vi "UHR-Fleezers Control (host) - 12.1_Jonathan.vi"() -> ()   [LabVIEW 2012] (continued)
            n1090 = Interleave 1D Arrays(w2555, w2554, w2553, w2538, w2552, w2551, w2501, w2521, w2520, w2500, w2519, w2518, w2523, w2522) -> (w2546:dbl[])
            n1091 = Divide(x=w2546, y=3276.7) -> (x/y=w2545:dbl[])
            n1092 = Decimate 1D Array(w2545) -> (w2544:dbl[], w2543:dbl[], w2542:dbl[], w2541:dbl[], w2540:dbl[], w2539:dbl[], w2497:dbl[], w2511:dbl[], w2495:dbl[], w2496:dbl[], w2509:dbl[], w2493:dbl[], w2507:dbl[], w2505:dbl[])
            n1093 = Negate(x=w2505) -> (-x=w2503:dbl[])
            n1094 = Divide(x=w2507, y=w2503) -> (x/y=w2506:dbl[])
            n1095 = Divide(x=w2496, y=w2493) -> (x/y=w2492:dbl[])
            n1096 = Divide(x=w2497, y=w2495) -> (x/y=w2494:dbl[])
            n1097 = Divide(x=w2544, y=w2542) -> (x/y=w2528:dbl[])
            n1098 = Divide(x=w2543, y=w2542) -> (x/y=w2527:dbl[])
            n1099 = Divide(x=w2541, y=w2539) -> (x/y=w2526:dbl[])
            n1100 = Divide(x=w2540, y=w2539) -> (x/y=w2525:dbl[])
            n1101 = Divide(x=w2511, y=w2495) -> (x/y=w2510:dbl[])
            n1102 = Divide(x=w2509, y=w2493) -> (x/y=w2508:dbl[])
            n1103 = Build Array(w2528, w2527, w2542, w2526, w2525, w2539, w2494, w2510, w2495, w2492, w2508, w2493, w2506, w2505) -> (w2504:dbl[][])
            n1104 = Bundle("T1 Y", "T1 X", "T1 Sum", "T2 Y", "T2 X", "T2 Sum", "T1 FB Y", "T1 FB X", "T1 FB Sum", "T2 FB Y", "T2 FB X", "T2 FB Sum", "PSD X", "PSD Y Sum") -> (w2491:T42)  [unwired: 1 out]
            n1105 = To Word Integer(number=w2546) -> (16bit integer=w2490:i16[])
            n1106 = Cluster To Array(cluster=w2491) -> (array=w2537:string[])
          }
        }
      }
    }
    "AI labels" <- w1624
    n1107 = Decimate 1D Array(w1598) -> (w1622:u32[], w1566:u32[])
    n1108 = local read "DMA Update Period (s)"() -> (w1634:dbl)
    n1109 = Build Array(w1622, w1566) -> (w1700:u32[][])
    n1110 = local read "Data Period (s)"() -> (w1472:dbl)
    n1111 = local read "BD 1 Frequency 2 (MHz)"() -> (w1505:dbl)
    n1112 = local read "BD 1 Frequency 1 (MHz)"() -> (w1506:dbl)
    n1113 = Decimate 1D Array(w1513) -> (w1537:i16[], w1536:i16[], w1534:i16[], w1533:i16[])  [unwired: 9 out]
    n1114 = To Double Precision Float(number=w1700) -> (double precision float=w1701:dbl[][])
    n1115 = local read "APD Integration Time (s)"() -> (w1579:dbl)
    n1116 = Multiply(x=w1472, y="Trap Pos. Disp. Downsample") -> (x*y=w1470:dbl)
    n1117 = Divide(x=w1537, y=w1536) -> (x/y=w1538:dbl[])
    n1118 = Divide(x=w1534, y=w1533) -> (x/y=w1535:dbl[])
    n1119 = feedback #6(0.0) -> (w1551:dbl)
    n1120 = Add(x=w1634, y=w1551) -> (x+y=w1740:dbl)
    n1121 = feedback-in #6(w1740) -> ()
    n1122 = local read "AOM X Cal (nm/MHz)"() -> (w1503:dbl)
    n1123 = To Time Stamp(1:w1551) -> (0:w1550:timestamp)
    n1124 = Split 1D Array(array=w1538, index="N El. to Ave.") -> (second subarray=w1541:dbl[])  [unwired: 1 out]
    n1125 = Split 1D Array(array=w1535, index="N El. to Ave.") -> (second subarray=w1540:dbl[])  [unwired: 1 out]
    n1126 = Multiply(x=w1472, y="Trap Disp. Downsample") -> (x*y=w1552:dbl)
    "Display Period (s)" <- w1552
    n1127 = for "Trap AI" {
      tunnel: [w2289] -> w1734 mode=indexing
      tunnel: w1550 -> [w2279]
      tunnel: "Trap Disp. Downsample" -> [w2287]
      tunnel: w1625 -> [w2285] mode=indexing
      tunnel: w1472 -> [w2284]
      tunnel: w1624 -> [w2283] mode=indexing
      tunnel: w1549 -> [w2282]
      tunnel: [w2281] -> w1590 mode=indexing
      tunnel: w1552 -> [w2280]
      workers-P: _ -> [_]
      n1128 = Bundle By Name("Y"=w2285, "dt"=w2284) -> (w2286:waveform(dbl))  [unwired: 1 out]
      n1129 = Set Waveform Attribute(5:w2283, 6:w2282, 7:w2286) -> (3:w2281:waveform(dbl))  [unwired: 1 in, 2 out]
      n1130 = call "downsample 1D array - double.vi"("Ave N"=w2287, "Array In"=w2285) -> ("Array Out"=w2288:dbl[])  [unwired: 1 out]
      n1131 = Bundle By Name(cluster=w2281, "t0"=w2279, "Y"=w2288, "dt"=w2280) -> (w2289:waveform(dbl))
    }
    n1132 = Bundle("BD 1 Frequency 1 (MHz)"=w1506, "BD 1 Frequency 2 (MHz)"=w1505) -> (w1507:T43)  [unwired: 1 out]
    n1133 = call-poly <vilib>:"Mean.vi"("X"=w1540) -> ("mean"=w1528:dbl)  [unwired: 1 out]
    n1134 = call-poly <vilib>:"Mean.vi"("X"=w1541) -> ("mean"=w1529:dbl)  [unwired: 1 out]
    n1135 = Reciprocal(x=w1552) -> (1/x=→"Trap Disp. Freq. (Hz)":dbl)
    n1136 = Cluster To Array(cluster=w1507) -> (array=w1504:dbl[])
    n1137 = local read "Trap X AI1 (DMA)"() -> (w1539:T14)
    n1138 = local read "Data points/scans (MCL)"() -> (w1712:dbl)
    n1139 = To Fixed-Point(number=w1528) -> (fixed-point=w1526:fxp<+/-,16,1>)  [unwired: 1 in]
    n1140 = To Fixed-Point(number=w1529) -> (fixed-point=w1527:fxp<+/-,16,1>)  [unwired: 1 in]
    n1141 = Bundle("Trap 1 Pos.", "Trap 2 Pos.") -> (w1548:cluster{string, string})  [unwired: 1 out]
    n1142 = Bundle By Name(cluster=w1539, "Set 1"=w1527, "Set 2"=w1526) -> (→"Trap X AI1 (DMA)":T14)
    n1143 = Cluster To Array(cluster=w1548) -> (array=w1545:string[])
    n1144 = Bundle("APD 1", "APD 2") -> (w1733:cluster{string, string})  [unwired: 1 out]
    n1145 = Select(t=-1.0, s="Negate Y Axis", f=1.0) -> (s? t:f=w1489:dbl)
    n1146 = for "Trap Position" {
      tunnel: w1554 -> [w1928] mode=indexing
      tunnel: "Trap Pos. Disp. Downsample" -> [w1927]
      tunnel: w1470 -> [w1925]
      tunnel: w1550 -> [w1924]
      tunnel: w1549 -> [w1922]
      tunnel: w1545 -> [w1921] mode=indexing
      tunnel: [w1920] -> w1459 mode=indexing
      tunnel: w1504 -> [w1918] mode=indexing
      tunnel: w1503 -> [w1916]
      tunnel: w1489 -> [w1915]
      n1147 = call "downsample 1D array - double.vi"("Ave N"=w1927, "Array In"=w1928) -> ("Array Out"=w1926:dbl[])  [unwired: 1 out]
      n1148 = Subtract(x=w1926, y=w1918) -> (x-y=w1919:dbl[])
      n1149 = Multiply(x=w1916, y=w1919) -> (x*y=w1917:dbl[])
      n1150 = Multiply(x=w1915, y=w1917) -> (x*y=w1914:dbl[])
      n1151 = Bundle By Name("Y"=w1914, "dt"=w1925, "t0"=w1924) -> (w1923:waveform(dbl))  [unwired: 1 out]
      n1152 = Set Waveform Attribute(5:w1921, 6:w1922, 7:w1923) -> (3:w1920:waveform(dbl))  [unwired: 1 in, 2 out]
    }
    n1153 = Cluster To Array(cluster=w1733) -> (array=w1730:string[])
    n1154 = for "APD" {
      tunnel: w1701 -> [w2268] mode=indexing
      tunnel: w1579 -> [w2276]
      tunnel: [w2272] -> w1586 mode=indexing
      tunnel: "APD Disp. Scale" -> [w2273]
      tunnel: w1549 -> [w2271]
      tunnel: w1730 -> [w2270] mode=indexing
      tunnel: "APD Disp. Downsample" -> [w2266]
      tunnel: [w2269] -> w1729
      workers-P: _ -> [_]
      tunnel: w1550 -> [w2265]
      n1155 = call "integrate 1D array interval - double.vi"("Ave N"=w2266, "Array In"=w2268) -> ("Array Out"=w2267:dbl[])  [unwired: 1 out]
      n1156 = Multiply(x=w2276, y=w2266) -> (x*y=w2269:dbl)
      n1157 = Divide(x=w2267, y=w2273) -> (x/y=w2274:dbl[])
      n1158 = Bundle By Name("t0"=w2265, "Y"=w2274, "dt"=w2269) -> (w2275:waveform(dbl))  [unwired: 1 out]
      n1159 = Set Waveform Attribute(5:w2270, 6:w2271, 7:w2275) -> (3:w2272:waveform(dbl))  [unwired: 1 in, 2 out]
    }
    "APD Display Period (s)" <- w1729
    n1160 = Reciprocal(x=w1729) -> (1/x=→"APD Display Freq. (Hz)":dbl)
    n1161 = local read "Display Period (s)"() -> (w1610:dbl)
    n1162 = Increment(x=w1712) -> (x+1=w1713:dbl)
    n1163 = To Double Precision Float(number=w1622) -> (double precision float=w1621:dbl[])
    n1164 = Index Array(array=w1459, index=0) -> (element=w1463:waveform(dbl))
    n1165 = Index Array(array=w1459, index=1) -> (element=w1458:waveform(dbl))
    n1166 = feedback #7(w1713) -> (w1716:dbl)
    n1167 = Select(t=0, s=w1703, f=w1716) -> (s? t:f=w1709:dbl)
    n1168 = Array Size(array=w1621) -> (size(s)=w1715:i32)
    n1169 = Add(x=w1715, y=w1709) -> (x+y=w1710:dbl)
    n1170 = Unbundle By Name(w1463) -> ("Y"=w1464:dbl[])
    n1171 = feedback #8(w1622) -> (w1699:u32[])
    n1172 = Build Array (concatenate)(w1699, w1622) -> (w1696:u32[])
    n1173 = feedback #9(w1566) -> (w1585:u32[])
    n1174 = Divide(x="Bead Sep. Int. Time (s)", y=w1610) -> (x/y=w1499:dbl)
    n1175 = Build Array (concatenate)(w1585, w1566) -> (w1584:u32[])
    n1176 = Add(x=w1464, y="FB Trap Pos Offset") -> (x+y=w1462:dbl[])
    "T1 x pos data" <- w1462
    n1177 = Greater?(x=w1710, y=w1712) -> (0:w1711:bool)
    n1178 = feedback #10(w1462) -> (w1501:dbl[])
    n1179 = Build Array (concatenate)(w1462, w1501) -> (w1500:dbl[])
    n1180 = Bundle By Name(cluster=w1463, "Y"=w1462) -> (w1461:waveform(dbl))
    n1181 = Select(t=w1709, s=w1711, f=w1710) -> (s? t:f=w1708:dbl)
    n1182 = feedback-in #7(w1708) -> ()
    n1183 = Array Size(array=w1696) -> (size(s)=w1693:i32)
    n1184 = Array Size(array=w1622) -> (size(s)=w1695:i32)
    n1185 = local read "MCL Scanning"() -> (w1706:bool)
    n1186 = local read "APD Integration Time (s)"() -> (w1593:dbl)
    n1187 = Bundle(w1461, w1458) -> (w1457:cluster{waveform(dbl), waveform(dbl)})  [unwired: 1 out]
    n1188 = Build Array (concatenate)(w1586, w1734) -> (w1588:waveform(dbl)[])
    "All Signals" <- w1588
    n1189 = Split 1D Array(array=w1500, index=w1499) -> (first subarray=w1493:dbl[])  [unwired: 1 out]
    n1190 = feedback-in #10(w1493) -> ()
    n1191 = Multiply(x=w1695, y="APD Ave N") -> (x*y=w1694:dbl)
    n1192 = Greater?(x=w1693, y=w1694) -> (0:w1697:bool)
    n1193 = Not(x=w1711) -> (.not. x?=w1705:bool)
    n1194 = Cluster To Array(cluster=w1457) -> (array=w1433:waveform(dbl)[])
    "Trap Positions" <- w1433
    n1195 = To Double Precision Float(number=w1566) -> (double precision float=w1565:dbl[])
    n1196 = call-poly <vilib>:"Mean.vi"("X"=w1493) -> ("mean"=w1492:dbl)  [unwired: 1 out]
    "Mean T1 Position (nm)" <- w1492
    n1197 = Subtract(x=w1493, y=w1492) -> (x-y=w1498:dbl[])
    n1198 = Square(x=w1498) -> (x^2=w1497:dbl[])
    n1199 = And(x=w1705, y=w1706) -> (x .and. y?=w1707:bool)
    n1200 = call-poly <vilib>:"Mean.vi"("X"=w1497) -> ("mean"=w1496:dbl)  [unwired: 1 out]
    n1201 = case shown="True" w1697 {
      tunnel: w1696 -> [w2048 w2055]
      tunnel: [w2048 w2053] -> w1639
      tunnel: w1694 -> [_ w2050]
      tunnel: w1693 -> [_ w2054]
      tunnel: w1584 -> [w2047 w2052]
      tunnel: [w2047 w2049] -> w1581
      frame False {
      }
      frame True {
        n1202 = Subtract(x=w2054, y=w2050) -> (x-y=w2051:dbl)
        n1203 = Array Subset(array=w2055, index=w2051, length=w2050) -> (w2053:u32[])
        n1204 = Array Subset(array=w2052, index=w2051, length=w2050) -> (w2049:u32[])
      }
    }
    n1205 = feedback-in #8(w1639) -> ()
    n1206 = feedback-in #9(w1581) -> ()
    n1207 = Square Root(x=w1496) -> (sqrt(x)=w1495:dbl)
    n1208 = Or(x=w1707, y=w1703) -> (x .or. y?=w1704:bool)
    n1209 = Equal?(x="Tab Control 6", y=T31."High Res Display") -> (x = y?=w1628:bool)
    n1210 = Multiply(x="APD Disp. Scale", y=w1586) -> (x*y=w1595:waveform(dbl)[])
    n1211 = Multiply(x=10.0, y=w1495) -> (x*y=→"Trap 1 Position RMS (A)":dbl)
    n1212 = Multiply(x="APD Disp. Downsample", y=w1593) -> (x*y=w1591:dbl)
    n1213 = Divide(x=w1595, y=w1591) -> (x/y=w1563:waveform(dbl)[])
    n1214 = case "For displaying the high resolution display (no downsampling)" shown="True" w1628 {
      tunnel: w1590 -> [_ w1948]
      frame False {
      }
      frame True {
        n1215 = Index Array(array=w1948, index="High Res. Display") -> (element=w1949:waveform(dbl))
        n1216 = call <vilib>:"Std Deviation and Variance.vi"("X"=w1949) -> ("mean"=w1956:dbl, "standard deviation"=w1961:dbl)  [unwired: 1 in, 1 out]
        "Mean Intensity" <- w1956
        "Sigma" <- w1961
        n1217 = Subtract(x=w1949, y=w1956) -> (x-y=w1955:waveform(dbl))
        n1218 = Select(t=w1955, s="Subtract mean", f=w1949) -> (s? t:f=→"1 Channel":waveform(dbl))
        n1219 = Divide(x=w1961, y=w1956) -> (x/y=→"Sigma/Mean":dbl)
        n1220 = feedback #11(1) -> (w1950:i32)
        n1221 = Greater Or Equal?(x=w1950, y="Slow mean N ave.") -> (x >= y?=w1963:bool)
        n1222 = Increment(x=w1950) -> (x+1=w1965:i32)
        n1223 = Select(t=1, s=w1963, f=w1965) -> (s? t:f=w1952:i32)
        n1224 = feedback-in #11(w1952) -> ()
        n1225 = feedback #12() -> (w1953:waveform(dbl))  [unwired: 1 out]
        n1226 = case shown="Default" w1950 {
          tunnel: [w1968 w1971] -> w1954
          tunnel: w1953 -> [w1970 _]
          tunnel: w1949 -> [w1969 w1971]
          frame Default {
            n1227 = call-poly <vilib>:"Append Waveforms.vi"("waveform B"=w1969, "waveform A"=w1970) -> ("waveform out"=w1968:waveform(dbl))  [unwired: 1 in, 8 out]
          }
          frame 1 {
          }
        }
        n1228 = feedback-in #12(w1954) -> ()
        n1229 = case shown="True" w1963 {
          tunnel: w1954 -> [_ w1967]
          frame False {
          }
          frame True {
            n1230 = call-poly <vilib>:"Mean.vi"("X"=w1967) -> ("mean"=→"Slow mean":dbl)  [unwired: 1 out]
          }
        }
      }
    }
    n1231 = Index Array(array=w1563, index=0) -> (element=w1573:waveform(dbl))
    n1232 = Index Array(array=w1563, index=1) -> (element=w1571:waveform(dbl))
    n1233 = case "For computing FFTs for display" shown="True" "Compute FFT" {
      tunnel: w1590 -> [_ w2662]
      frame False {
      }
      frame True {
        n1234 = Build Array("FFT 1 Choice 1", "FFT 1 Choice 2", "FFT 2 Choice 1", "FFT 2 Choice 2") -> (w2655:u16[])
        n1235 = Array Size(array=w2662) -> (size(s)=w2661:i32)
        n1236 = feedback-in #13(w2655) -> ()
        n1237 = feedback #13(u16[] [100, 100, 100, 100]) -> (w2656:u16[])
        n1238 = feedback-in #14("# Spectra to Ave.") -> ()
        n1239 = feedback #14("# Spectra to Ave.") -> (w2653:dbl)
        n1240 = Not Equal?(x="# Spectra to Ave.", y=w2653) -> (x != y?=w2652:bool)
        n1241 = Not Equal?(x=w2655, y=w2656) -> (x != y?=w2654:bool)
        n1242 = feedback #15(1.0) -> (w2639:dbl)
        n1243 = Compound Arithmetic op=OR("Reset FFT", w2654, w2652) -> (w2637:bool)
        n1244 = Select(t=1.0, s=w2637, f=w2639) -> (s? t:f=w2641:dbl)
        n1245 = Greater?(x=w2641, y="# Spectra to Ave.") -> (0:w2660:bool)
        n1246 = Increment(x=w2641) -> (x+1=w2640:dbl)
        n1247 = feedback-in #15(w2640) -> ()
        n1248 = local read "DMA Update Period (s)"() -> (w2635:dbl)
        n1249 = Multiply(x="# Spectra to Ave.", y=w2635) -> (x*y=→"Ave. Time (s)":dbl)
        n1250 = Build Array(cluster{"f0":dbl, "df":dbl, "magnitude":dbl[]} {"f0"=0.0, "df"=0.0, "magnitude"=[]} ("PSD")) -> (w2644:cluster{"f0":dbl, "df":dbl, "magnitude":dbl[]}[])
        n1251 = Build Array(w2644, w2644, w2644, w2644) -> (w2646:T44)
        n1252 = feedback #16(w2646) -> (w2651:T44)
        n1253 = for {
          N: 4 -> [_]
          tunnel: w2655 -> [w2684] mode=indexing
          tunnel: w2662 -> [w2685]
          tunnel: w2661 -> [w2687]
          tunnel: w2637 -> [w2680]
          tunnel: w2660 -> [w2679]
          tunnel: "# Spectra to Ave." -> [w2678]
          tunnel: [w2677] -> w2650 mode=indexing
          tunnel: w2651 -> [w2682] mode=indexing
          tunnel: [w2681] -> w2638 mode=indexing
          tunnel: w2641 -> [w2676]
          n1254 = Less?(x=w2684, y=w2687) -> (x < y?=w2686:bool)
          n1255 = Index Array(array=w2685, index=w2684) -> (element=w2683:waveform(dbl))
          n1256 = case shown="True" w2686 {
            tunnel: w2683 -> [_ w2704]
            tunnel: w2682 -> [w2689 w2702]
            tunnel: [w2689 w2690] -> w2681
            tunnel: w2680 -> [_ w2701]
            tunnel: w2679 -> [_ w2694]
            tunnel: w2678 -> [_ w2693]
            tunnel: [cluster{"f0":dbl, "df":dbl, "magnitude":dbl[]} {"f0"=0.0, "df"=0.0, "magnitude"=[]} ("PSD") w2695] -> w2677
            tunnel: w2676 -> [_ w2692]
            frame False {
            }
            frame True {
              n1257 = call <vilib>:"Std Deviation and Variance.vi"("X"=w2704) -> ("mean"=w2705:dbl)  [unwired: 1 in, 2 out]
              n1258 = Subtract(x=w2704, y=w2705) -> (x-y=w2703:waveform(dbl))
              n1259 = xnode "Spectral Measurements"("Signals"=w2703) -> ("PSD"=w2697:cluster{"f0":dbl, "df":dbl, "magnitude":dbl[]})  [unwired: 1 in, 1 out]
              n1260 = case shown="False" w2701 {
                tunnel: w2702 -> [w2714 _]
                tunnel: [w2710 w2719] -> w2690
                tunnel: w2697 -> [w2713 w2720]
                tunnel: w2694 -> [w2712 _]
                frame False {
                  n1261 = Build Array (concatenate)(w2714, w2713) -> (w2711:cluster{"f0":dbl, "df":dbl, "magnitude":dbl[]}[])
                  n1262 = case shown="True" w2712 {
                    tunnel: w2711 -> [w2715 w2718]
                    tunnel: [w2715 w2716] -> w2710
                    frame False {
                    }
                    frame True {
                      n1263 = Delete From Array(array=w2718, index=0) -> (array with subset deleted=w2716:cluster{"f0":dbl, "df":dbl, "magnitude":dbl[]}[])  [unwired: 1 in, 1 out]
                    }
                  }
                }
                frame True {
                  n1264 = Build Array(w2720) -> (w2719:cluster{"f0":dbl, "df":dbl, "magnitude":dbl[]}[])
                }
              }
              n1265 = for {
                tunnel: w2690 -> [w2709] mode=indexing
                tunnel: [w2708] -> w2700 mode=indexing
                workers-P: _ -> [_]
                n1266 = Unbundle By Name(w2709) -> ("magnitude"=w2708:dbl[])
              }
              n1267 = Transpose 2D Array(2D array=w2700) -> (transposed array=w2699:dbl[][])
              n1268 = for {
                tunnel: w2699 -> [w2707] mode=indexing
                tunnel: [w2706] -> w2698 mode=indexing
                workers-P: _ -> [_]
                n1269 = Add Array Elements(numeric array=w2707) -> (sum=w2706:dbl)
              }
              n1270 = Select(t=w2693, s=w2694, f=w2692) -> (s? t:f=w2691:dbl)
              n1271 = Divide(x=w2698, y=w2691) -> (x/y=w2696:dbl[])
              n1272 = Bundle By Name(cluster=w2697, "magnitude"=w2696) -> (w2695:cluster{"f0":dbl, "df":dbl, "magnitude":dbl[]})
            }
          }
        }
        n1273 = case shown="True" w2637 {
          tunnel: w2638 -> [w2669 w2675]
          tunnel: [w2669 w2670] -> w2636
          frame False {
          }
          frame True {
            n1274 = Array Subset(array=w2675, index (row)=0 ("index"), length (row)=4 ("length"), index (col)=0 ("index"), length (col)=1 ("length")) -> (w2670:T44)
          }
        }
        n1275 = feedback-in #16(w2636) -> ()
        n1276 = Split 1D Array(array=w2650, index=2) -> (first subarray=→"FFT 1":cluster{"f0":dbl, "df":dbl, "magnitude":dbl[]}[], second subarray=→"FFT 2":cluster{"f0":dbl, "df":dbl, "magnitude":dbl[]}[])
      }
    }
    n1277 = case "For plotting results of scanning MCL" shown="True" w1704 {
      tunnel: w1703 -> [_ w2088]
      tunnel: w1621 -> [_ w2184]
      tunnel: w1712 -> [_ _]
      tunnel: w1590 -> [_ w2158]
      tunnel: w1565 -> [_ w2089]
      tunnel: w1564 -> [_ w2062]
      frame False {
      }
      frame True {
        w2069 = u32 0 items=["Horizontal", "Vertical", "Central", "1st Diagonal", "2nd Diagonal"] ("Type of Symmetry")
        w2097 = u32 0 items=["Horizontal", "Vertical", "Central", "1st Diagonal", "2nd Diagonal"] ("Type of Symmetry")
        w2100 = u32 0 items=["Horizontal", "Vertical", "Central", "1st Diagonal", "2nd Diagonal"] ("Type of Symmetry")
        w2129 = u32 0 items=["Horizontal", "Vertical", "Central", "1st Diagonal", "2nd Diagonal"] ("Type of Symmetry")
        n1278 = Index Array(array=w2158, index=10) -> (element=w2164:waveform(dbl))
        n1279 = Index Array(array=w2158, index=11) -> (element=w2161:waveform(dbl))
        n1280 = local read "Cycles/step (MCL)"() -> (w2114:u64)
        n1281 = Index Array(array=w2158, index="Channel") -> (element=w2160:waveform(dbl))
        n1282 = Unbundle(w2062) -> ("New Image"=w2061:T3, "New Image"=w2060:T3, "New Image"=w2059:T3, "New Image"=w2058:T3)
        n1283 = Unbundle By Name(w2164) -> ("Y"=w2116:dbl[])
        n1284 = Unbundle By Name(w2161) -> ("Y"=w2118:dbl[])
        n1285 = Unbundle By Name(w2160) -> ("Y"=w2123:dbl[])
        n1286 = call "downsample 1D array - double.vi"("Ave N"=w2114, "Array In"=w2116) -> ("Array Out"=w2115:dbl[])  [unwired: 1 out]
        n1287 = call "downsample 1D array - double.vi"("Ave N"=w2114, "Array In"=w2118) -> ("Array Out"=w2117:dbl[])  [unwired: 1 out]
        n1288 = call "downsample 1D array - double.vi"("Ave N"=w2114, "Array In"=w2123) -> ("Array Out"=w2122:dbl[])  [unwired: 1 out]
        n1289 = feedback #17(w2184) -> (w2185:dbl[])
        n1290 = Build Array (concatenate)(w2185, w2184) -> (w2166:dbl[])
        n1291 = feedback #18(w2089) -> (w2091:dbl[])
        n1292 = Build Array (concatenate)(w2091, w2089) -> (w2090:dbl[])
        n1293 = local read "Scan steps (MCL)"() -> (w2071:u64)
        n1294 = Select(t=w2184, s=w2088, f=w2166) -> (s? t:f=w2170:dbl[])
        n1295 = feedback-in #17(w2170) -> ()
        n1296 = Select(t=w2089, s=w2088, f=w2090) -> (s? t:f=w2072:dbl[])
        n1297 = feedback-in #18(w2072) -> ()
        n1298 = local read "Scan lines (y)"() -> (w2057:u64)
        n1299 = local read "N APD Samp/step"() -> (w2073:dbl)
        n1300 = feedback #19(w2115) -> (w2172:dbl[])
        n1301 = Build Array (concatenate)(w2172, w2115) -> (w2163:dbl[])
        n1302 = feedback #20(w2122) -> (w2182:dbl[])
        n1303 = Build Array (concatenate)(w2182, w2122) -> (w2181:dbl[])
        n1304 = feedback #21(w2117) -> (w2174:dbl[])
        n1305 = Build Array (concatenate)(w2174, w2117) -> (w2175:dbl[])
        n1306 = Select(t=w2115, s=w2088, f=w2163) -> (s? t:f=w2119:dbl[])
        n1307 = feedback-in #19(w2119) -> ()
        n1308 = Select(t=w2122, s=w2088, f=w2181) -> (s? t:f=w2121:dbl[])
        n1309 = feedback-in #20(w2121) -> ()
        n1310 = Select(t=w2117, s=w2088, f=w2175) -> (s? t:f=w2120:dbl[])
        n1311 = feedback-in #21(w2120) -> ()
        n1312 = Multiply(x=w2071, y=u64 2) -> (x*y=w2056:u64)
        n1313 = call "integrate 1D array interval - double.vi"("Ave N"=w2073, "Array In"=w2072) -> ("Array Out"=w2084:dbl[])  [unwired: 1 out]
        n1314 = call "integrate 1D array interval - double.vi"("Ave N"=w2073, "Array In"=w2170) -> ("Array Out"=w2169:dbl[])  [unwired: 1 out]
        n1315 = Array Size(array=w2084) -> (size(s)=w2085:i32)
        n1316 = Array Size(array=w2169) -> (size(s)=w2171:i32)
        n1317 = Multiply(x=w2057, y=w2056) -> (x*y=w2087:u64)
        n1318 = Multiply(x=w2057, y=w2056) -> (x*y=w2179:u64)
        n1319 = call-poly <vilib>:"Mean.vi"("X"=w2119) -> ("mean"=w2103:dbl)  [unwired: 1 out]
        n1320 = Subtract(x=w2087, y=w2085) -> (x-y=w2078:u64)
        n1321 = call-poly <vilib>:"Mean.vi"("X"=w2121) -> ("mean"=w2108:dbl)  [unwired: 1 out]
        n1322 = call-poly <vilib>:"Mean.vi"("X"=w2120) -> ("mean"=w2106:dbl)  [unwired: 1 out]
        n1323 = call-poly <vilib>:"Mean.vi"("X"=w2084) -> ("mean"=w2075:dbl)  [unwired: 1 out]
        n1324 = Subtract(x=w2179, y=w2171) -> (x-y=w2113:u64)
        n1325 = call-poly <vilib>:"Mean.vi"("X"=w2169) -> ("mean"=w2110:dbl)  [unwired: 1 out]
        n1326 = Initialize Array(1.0 ("element"), w2078) -> (w2074:dbl[])
        n1327 = Initialize Array(1.0 ("element"), w2113) -> (w2104:dbl[])
        n1328 = Multiply(x=w2074, y=w2075) -> (x*y=w2076:dbl[])
        n1329 = Multiply(x=w2104, y=w2106) -> (x*y=w2107:dbl[])
        n1330 = Multiply(x=w2104, y=w2108) -> (x*y=w2109:dbl[])
        n1331 = Multiply(x=w2104, y=w2103) -> (x*y=w2105:dbl[])
        n1332 = Multiply(x=w2104, y=w2110) -> (x*y=w2111:dbl[])
        n1333 = Build Array (concatenate)(w2119, w2105) -> (w2173:dbl[])
        n1334 = Build Array (concatenate)(w2121, w2109) -> (w2177:dbl[])
        n1335 = Build Array (concatenate)(w2120, w2107) -> (w2176:dbl[])
        n1336 = Build Array (concatenate)(w2084, w2076) -> (w2086:dbl[])
        n1337 = Build Array (concatenate)(w2169, w2111) -> (w2178:dbl[])
        n1338 = Reshape Array(w2173, w2057, w2056) -> (w2139:dbl[][])
        n1339 = Reshape Array(w2086, w2057, w2056) -> (w2082:dbl[][])
        n1340 = Reshape Array(w2177, w2057, w2056) -> (w2131:dbl[][])
        n1341 = Reshape Array(w2176, w2057, w2056) -> (w2146:dbl[][])
        n1342 = Reshape Array(w2178, w2057, w2056) -> (w2156:dbl[][])
        n1343 = Array Subset(array=w2146, index (col)=0 ("index"), length (col)=w2071) -> (w2151:dbl[][])  [unwired: 2 in]
        n1344 = Array Subset(array=w2146, index (col)=w2071) -> (w2149:dbl[][])  [unwired: 3 in]
        n1345 = Array Subset(array=w2131, index (col)=0 ("index"), length (col)=w2071) -> (w2137:dbl[][])  [unwired: 2 in]
        n1346 = Array Subset(array=w2131, index (col)=w2071) -> (w2135:dbl[][])  [unwired: 3 in]
        n1347 = Array Subset(array=w2082, index (col)=0 ("index"), length (col)=w2071) -> (w2081:dbl[][])  [unwired: 2 in]
        n1348 = Array Subset(array=w2082, index (col)=w2071) -> (w2079:dbl[][])  [unwired: 3 in]
        n1349 = Array Subset(array=w2156, index (col)=0 ("index"), length (col)=w2071) -> (w2155:dbl[][])  [unwired: 2 in]
        n1350 = Array Subset(array=w2156, index (col)=w2071) -> (w2153:dbl[][])  [unwired: 3 in]
        n1351 = Array Subset(array=w2139, index (col)=0 ("index"), length (col)=w2071) -> (w2144:dbl[][])  [unwired: 2 in]
        n1352 = Array Subset(array=w2139, index (col)=w2071) -> (w2142:dbl[][])  [unwired: 3 in]
        n1353 = for {
          tunnel: w2151 -> [w2193] mode=indexing
          tunnel: [w2192] -> w2150 mode=indexing
          workers-P: _ -> [_]
          n1354 = Reverse 1D Array(array=w2193) -> (reversed array=w2192:dbl[])
        }
        n1355 = for {
          tunnel: w2137 -> [w2189] mode=indexing
          tunnel: [w2188] -> w2136 mode=indexing
          workers-P: _ -> [_]
          n1356 = Reverse 1D Array(array=w2189) -> (reversed array=w2188:dbl[])
        }
        n1357 = for {
          tunnel: w2081 -> [w2187] mode=indexing
          tunnel: [w2186] -> w2080 mode=indexing
          workers-P: _ -> [_]
          n1358 = Reverse 1D Array(array=w2187) -> (reversed array=w2186:dbl[])
        }
        n1359 = for {
          tunnel: w2155 -> [w2195] mode=indexing
          tunnel: [w2194] -> w2154 mode=indexing
          workers-P: _ -> [_]
          n1360 = Reverse 1D Array(array=w2195) -> (reversed array=w2194:dbl[])
        }
        n1361 = for {
          tunnel: w2144 -> [w2191] mode=indexing
          tunnel: [w2190] -> w2143 mode=indexing
          workers-P: _ -> [_]
          n1362 = Reverse 1D Array(array=w2191) -> (reversed array=w2190:dbl[])
        }
        n1363 = Index Array(array=w2156, index (row)=0) -> (element=→"Waveform Graph":dbl[])  [unwired: 1 in]
        n1364 = Add(x=w2150, y=w2149) -> (x+y=w2148:dbl[][])
        n1365 = Add(x=w2136, y=w2135) -> (x+y=w2134:dbl[][])
        n1366 = Add(x=w2080, y=w2079) -> (x+y=w2064:dbl[][])
        n1367 = Add(x=w2154, y=w2153) -> (x+y=w2128:dbl[][])
        n1368 = Add(x=w2143, y=w2142) -> (x+y=w2141:dbl[][])
        n1369 = Divide(x=w2134, y=2) -> (x/y=w2132:dbl[][])
        n1370 = Divide(x=w2148, y=2) -> (x/y=w2093:dbl[][])
        n1371 = Divide(x=w2141, y=2) -> (x/y=w2095:dbl[][])
        n1372 = To Single Precision Float(number=w2128) -> (single precision float=w2127:sgl[][])
        n1373 = Transpose 2D Array(2D array=w2132) -> (transposed array=→"Data map":dbl[][])
        n1374 = To Single Precision Float(number=w2064) -> (single precision float=w2068:sgl[][])
        n1375 = To Single Precision Float(number=w2093) -> (single precision float=w2099:sgl[][])
        n1376 = To Single Precision Float(number=w2095) -> (single precision float=w2096:sgl[][])
        n1377 = call "IMAQ ArrayToImage"("Image Pixels (Float)"=w2127, "Image"=w2061) -> ("Image Out"=w2130:T3)  [unwired: 8 in, 1 out]
        n1378 = call "IMAQ ArrayToImage"("Image Pixels (Float)"=w2068, "Image"=w2060) -> ("Image Out"=w2070:T3)  [unwired: 8 in, 1 out]
        n1379 = call "IMAQ ArrayToImage"("Image Pixels (Float)"=w2099, "Image"=w2059) -> ("Image Out"=w2101:T3)  [unwired: 8 in, 1 out]
        n1380 = call "IMAQ ArrayToImage"("Image Pixels (Float)"=w2096, "Image"=w2058) -> ("Image Out"=w2098:T3)  [unwired: 8 in, 1 out]
        n1381 = call "IMAQ Symmetry"("Type of Symmetry"=w2129, "Image Src"=w2130) -> ("Image Dst Out"=w2125:T3)  [unwired: 3 in, 1 out]
        n1382 = call "IMAQ Symmetry"("Type of Symmetry"=w2069, "Image Src"=w2070) -> ("Image Dst Out"=w2066:T3)  [unwired: 3 in, 1 out]
        n1383 = call "IMAQ Symmetry"("Type of Symmetry"=w2100, "Image Src"=w2101) -> ("Image Dst Out"=→"Detection Laser X":T3)  [unwired: 3 in, 1 out]
        n1384 = call "IMAQ Symmetry"("Type of Symmetry"=w2097, "Image Src"=w2098) -> ("Image Dst Out"=→"Detection Laser Y":T3)  [unwired: 3 in, 1 out]
        n1385 = call "IMAQ Set Simple Calibration"("Calibration Axis Info"=T32 {"Origin Pixel"={"X"=0.0, "Y"=0.0}, "Angle Relative to Horizontal (deg)"=0.0, "Axis Reference"=0}, "Grid Descriptor"=T33 {"X Step"=0.3, "Y Step"=0.3, "Unit"=enum."Undefined"}, "Image"=w2125) -> ("Calibrated Image"=→"APD 1":T3)  [unwired: 7 in, 1 out]
        n1386 = call "IMAQ Set Simple Calibration"("Calibration Axis Info"=T32 {"Origin Pixel"={"X"=0.0, "Y"=0.0}, "Angle Relative to Horizontal (deg)"=0.0, "Axis Reference"=0}, "Grid Descriptor"=T33 {"X Step"=0.3, "Y Step"=0.3, "Unit"=enum."Undefined"}, "Image"=w2066) -> ("Calibrated Image"=→"APD 2":T3)  [unwired: 7 in, 1 out]
      }
    }
    n1387 = Subtract(x=w1571, y="APD 2 Offset") -> (x-y=w1568:waveform(dbl))
    n1388 = Subtract(x=w1573, y="APD 1 Offset") -> (x-y=w1569:waveform(dbl))
    n1389 = Index Array(array=w1588, index=3) -> (element=w1648:waveform(dbl))
    n1390 = Index Array(array=w1588, index=6) -> (element=w1645:waveform(dbl))
    n1391 = Build Array(w1569, w1568) -> (→"APD Chart":waveform(dbl)[])
    n1392 = Array Size(array=w1639) -> (size(s)=w1692:i32)
    n1393 = call <vilib>:"Std Deviation and Variance.vi"("X"=w1581) -> ("standard deviation"=w1580:dbl)  [unwired: 1 in, 2 out]
    n1394 = Add Array Elements(numeric array=w1581) -> (sum=w1583:u32)
    n1395 = Add Array Elements(numeric array=w1639) -> (sum=w1702:u32)
    n1396 = call <vilib>:"Std Deviation and Variance.vi"("X"=w1639) -> ("standard deviation"=w1638:dbl)  [unwired: 1 in, 2 out]
    n1397 = Divide(x="T1 offset_x (mV)", y=1000.0) -> (x/y=w1649:dbl)
    n1398 = Divide(x=w1580, y=w1579) -> (x/y=w1576:dbl)
    "Rate sigma (Hz) 2" <- w1576
    n1399 = Multiply(x=w1579, y=w1692) -> (x*y=w1582:dbl)
    "Int. Time (s)" <- w1582
    n1400 = Divide(x=w1583, y=w1582) -> (x/y=w1577:dbl)
    "APD 2 Rate (Hz)" <- w1577
    n1401 = Divide(x=w1702, y=w1582) -> (x/y=w1636:dbl)
    "APD 1 Rate (Hz)" <- w1636
    n1402 = Divide(x=w1638, y=w1579) -> (x/y=w1637:dbl)
    "Rate sigma (Hz)" <- w1637
    n1403 = Divide(x=w1576, y=w1577) -> (x/y=→"Sigma/Mean 2":dbl)
    n1404 = Divide(x=w1637, y=w1636) -> (x/y=→"Sigma/Mean":dbl)
    n1405 = feedback-in #22("Calibration") -> ()
    n1406 = feedback #22(u16 1 ("Calibration")) -> (w1669:u16)
    n1407 = Divide(x="T2 offset_x (mV)", y=1000.0) -> (x/y=w1647:dbl)
    n1408 = case shown="0, Default" "Calibration" {
      tunnel: "T1 alpha_x (nm/V)" -> [_ w2024 w2045]
      tunnel: "T1 kappa_x (pN/nm)" -> [_ _ w2035]
      tunnel: "T2 alpha_x (nm/V)" -> [_ w2023 w2043]
      tunnel: "T2 kappa_x (pN/nm)" -> [_ _ w2036]
      tunnel: w1648 -> [w2006 w2021 w2041]
      tunnel: w1645 -> [w2005 w2019 w2039]
      tunnel: [w2006 w2018 w2038] -> w1678
      tunnel: [w2005 w2017 w2037] -> w1677
      tunnel: ["T1 X (V)" ("Label.Text") "T1 X (nm)" ("Label.Text") "T1 X (pN)" ("Label.Text")] -> w1666
      tunnel: ["T2 X (V)" ("Label.Text") "T2 X (nm)" ("Label.Text") "T2 X (pN)" ("Label.Text")] -> w1665
      tunnel: ["Position (V)" ("Label.Text") "Position (nm)" ("Label.Text") "Force (pN)" ("Label.Text")] -> w1667
      tunnel: w1647 -> [_ w2009 w2028]
      tunnel: w1649 -> [_ w2012 w2030]
      tunnel: ["Mean (V)" ("Label.Text") "Mean (nm)" ("Label.Text") "Mean (pN)" ("Label.Text")] -> w1662
      tunnel: ["Difference (V)" ("Label.Text") "Difference (nm)" ("Label.Text") "Difference (pN)" ("Label.Text")] -> w1596
      frame 0, Default {
      }
      frame 1 {
        n1409 = Unbundle By Name(w2021) -> ("Y"=w2025:dbl[])
        n1410 = Unbundle By Name(w2019) -> ("Y"=w2010:dbl[])
        n1411 = Subtract(x=w2025, y=w2012) -> (x-y=w2013:dbl[])
        n1412 = Subtract(x=w2010, y=w2009) -> (x-y=w2011:dbl[])
        n1413 = Multiply(x=w2011, y=w2023) -> (x*y=w2020:dbl[])
        n1414 = Multiply(x=w2024, y=w2013) -> (x*y=w2022:dbl[])
        n1415 = Bundle By Name(cluster=w2019, "Y"=w2020) -> (w2017:waveform(dbl))
        n1416 = Bundle By Name(cluster=w2021, "Y"=w2022) -> (w2018:waveform(dbl))
      }
      frame 2 {
        n1417 = Unbundle By Name(w2041) -> ("Y"=w2046:dbl[])
        n1418 = Unbundle By Name(w2039) -> ("Y"=w2044:dbl[])
        n1419 = Subtract(x=w2044, y=w2028) -> (x-y=w2029:dbl[])
        n1420 = Subtract(x=w2046, y=w2030) -> (x-y=w2031:dbl[])
        n1421 = Compound Arithmetic op=MULTIPLY(w2029, w2043, w2036) -> (w2040:dbl[])
        n1422 = Compound Arithmetic op=MULTIPLY(w2035, w2045, w2031) -> (w2042:dbl[])
        n1423 = Bundle By Name(cluster=w2039, "Y"=w2040) -> (w2037:waveform(dbl))
        n1424 = Bundle By Name(cluster=w2041, "Y"=w2042) -> (w2038:waveform(dbl))
      }
    }
    n1425 = Not Equal?(x=w1669, y="Calibration") -> (x != y?=w1626:bool)
    n1426 = case shown="True" w1626 {
      tunnel: w1667 -> [_ w1999]
      tunnel: w1666 -> [_ w1998]
      tunnel: w1665 -> [_ w1997]
      tunnel: w1662 -> [_ w1996]
      tunnel: w1596 -> [_ w1995]
      frame False {
      }
      frame True {
        n1427 = property on="Force" class="WFChart (strict)"("YScale.NameLbl.Text"=w1999) -> ()  [unwired: 2 in, 2 out]
        n1428 = property on="T2 X" class="DigNum (strict)"("Caption.Text"=w1997) -> ()  [unwired: 2 in, 2 out]
        n1429 = property on="T1 X" class="DigNum (strict)"("Caption.Text"=w1998) -> ()  [unwired: 2 in, 2 out]
        n1430 = property on="Mean" class="DigNum (strict)"("Caption.Text"=w1996) -> ()  [unwired: 2 in, 2 out]
        n1431 = property on="Difference" class="DigNum (strict)"("Caption.Text"=w1995) -> ()  [unwired: 2 in, 2 out]
      }
    }
    n1432 = Unbundle By Name(w1648) -> ("Y"=w1651:dbl[])
    n1433 = Unbundle By Name(w1645) -> ("Y"=w1654:dbl[])
    n1434 = Subtract(x=w1651, y=w1649) -> (x-y=w1652:dbl[])
    n1435 = Subtract(x=w1654, y=w1647) -> (x-y=w1653:dbl[])
    n1436 = Multiply(x=w1653, y="T2 alpha_x (nm/V)") -> (x*y=w1438:dbl[])
    n1437 = Multiply(x="T1 alpha_x (nm/V)", y=w1652) -> (x*y=w1439:dbl[])
    n1438 = Not(x="Trap Trig. Fl.") -> (.not. x?=w1475:bool)
    n1439 = Multiply(x=w1677, y=-1.0) -> (x*y=w1656:waveform(dbl))
    n1440 = Subtract(x=w1439, y=w1438) -> (x-y=w1644:dbl[])
    n1441 = Unbundle By Name(w1677) -> ("Y"=w1615:dbl[])
    n1442 = Unbundle By Name(w1678) -> ("Y"=w1440:dbl[])
    n1443 = Negate(x=w1644) -> (-x=w1436:dbl[])
    n1444 = Build Array(w1678, w1656) -> (→"Force":waveform(dbl)[])
    n1445 = Subtract(x=w1436, y="Offset (nm)") -> (x-y=w1613:dbl[])
    n1446 = case shown="True" "Read Lateness and Rel Phase" {
      tunnel: w1456 -> [w1972 w1994]
      tunnel: w1455 -> [w1973 w1993]
      tunnel: [w1972 w1992] -> w1642
      tunnel: [w1973 w1991] -> w1641
      frame False {
      }
      frame True {
        n1447 = xnode "Read/Write Control"("FPGA VI Reference In"=w1994, "error in"=w1993) -> ("FPGA VI Reference Out"=w1992:T20, "error out"=w1991:errorcluster, "GI Relative phase"=→"GI relative phase":i16, "Relative phase"=→"Relative phase (AI1)":i16, "AI Late Counter"=→"Late Counter (AI1)":u16, "GI Late Counter"=→"GI Late Counter":u16, "MCL Late Counter"=→"MCL Late Counter":u16, "MCL Relative Phase"=→"Relative Phase (MCL)":i16, "APD Acq Relative Phase"=→"APD Acq Relative Phase":i16, "APD 1 Gate Relative Phase"=→"APD 1 Gate Relative Phase":i16, "APD 2 Gate Relative Phase"=→"APD 2 Gate Relative Phase":i16, "APD Acq Late Counter"=→"APD Acq Late Counter":u16, "APD 1 Gate Late Counter"=→"APD 1 Gate Late Counter":u16, "APD 2 Gate Late Counter"=→"APD 2 Gate Late Counter":u16, "Green FB Relative Phase"=→"Relative phase (Green FB)":i16, "GI Relative phase 2"=→"GI relative phase 2":i16, "GI Late Counter 2"=→"GI Late Counter 2":u16, "Trap Pos FIFO Timeout"=→"Trap Pos FIFO Timeout":u16, "Trap AI FIFO Timeout"=→"Trap AI FIFO Timeout":u16)
      }
    }
    n1448 = call-poly <vilib>:"Mean.vi"("X"=w1615) -> ("mean"=w1442:dbl)  [unwired: 1 out]
    "T2 X" <- w1442
    n1449 = Negate(x=w1615) -> (-x=w1616:dbl[])
    n1450 = call-poly <vilib>:"Mean.vi"("X"=w1440) -> ("mean"=w1443:dbl)  [unwired: 1 out]
    "T1 X" <- w1443
    n1451 = Negate(x=w1442) -> (-x=w1441:dbl)
    n1452 = Bundle By Name(cluster=w1648, "Y"=w1613) -> (w1587:waveform(dbl))
    "Bead Separation" <- w1587
    n1453 = Add(x=w1440, y=w1616) -> (x+y=w1617:dbl[])
    n1454 = Add(x=w1443, y=w1441) -> (x+y=w1664:dbl)
    n1455 = Subtract(x=w1443, y=w1441) -> (x-y=→"Difference":dbl)
    n1456 = Divide(x=w1617, y=2.0) -> (x/y=→"Vec Mean of T1 T2":dbl[])
    n1457 = Divide(x=w1664, y=2.0) -> (x/y=w1619:dbl)
    "Mean" <- w1619
    n1458 = feedback-in #23("Trap Trig. Fl.") -> ()
    n1459 = feedback #23("Trap Trig. Fl.") -> (w1473:bool)
    n1460 = And(x=w1475, y=w1473) -> (x .and. y?=w1474:bool)
    n1461 = case "If have just turned off triggering" shown="True" w1474 {
      tunnel: w1456 -> [_ w1807]
      tunnel: w1455 -> [_ w1806]
      frame False {
      }
      frame True {
        w1805 = FALSE ("FPGA Trap Trig")
        n1462 = xnode "Read/Write Control"("FPGA VI Reference In"=w1807, "error in"=w1806, "FPGA Trap Trig"=w1805) -> ("FPGA VI Reference Out"=w1804:T20, "error out"=w1803:errorcluster)
        n1463 = xnode "Read/Write Control"("FPGA VI Reference In"=w1804, "error in"=w1803, "TTrig?"=w1805) -> ()  [unwired: 2 out]
        n1464 = local write "Initializing"(FALSE ("Initializing")) -> ()
        n1465 = local write "Triggered"(FALSE ("Triggered")) -> ()
        n1466 = local write "Waiting"(FALSE ("Waiting")) -> ()
      }
    }
    n1467 = Not(x=w1473) -> (.not. x?=w1486:bool)
    n1468 = And(x="Trap Trig. Fl.", y=w1486) -> (x .and. y?=w1483:bool)
    n1469 = local read "Tether"() -> (w1620:bool)
    n1470 = Or(x=w1483, y="Reinitialize") -> (x .or. y?=w1469:bool)
    n1471 = feedback #24(w1479) -> (w1484:string)
    n1472 = Select(t=w1479, s=w1483, f=w1484) -> (s? t:f=w1478:string)
    n1473 = Select(t=w1479, s="Reinitialize", f=w1478) -> (s? t:f=w1477:string)
    n1474 = feedback #25(0) -> (w1481:i32)
    n1475 = feedback #26(w1613) -> (w1612:dbl[])
    n1476 = Build Array (concatenate)(w1613, w1612) -> (w1437:dbl[])
    n1477 = case "For determining if there is a tether still" shown="True" w1620 {
      tunnel: w1619 -> [_ w1931]
      frame False {
      }
      frame True {
        n1478 = Greater?(x="Lost Tether Alarm Threshold (pN)", y=w1931) -> (0:w1929:bool)
        n1479 = case shown="True" w1929 {
          frame False {
          }
          frame True {
            w1932 = FALSE ("Value (Signaling)")
            n1480 = flat-sequence {
              frame #0 {
                # "stop only if saving"
                n1481 = local read "Saving..."() -> (w1944:bool)
                n1482 = And(x=w1944, y="TA Cancel Save?") -> (x .and. y?=w1943:bool)
                n1483 = local write "Stop Saving"(w1943) -> ()
              }
              frame #1 {
                n1484 = case shown="True" "TA Green Off?" {
                  frame False {
                  }
                  frame True {
                    w1947 = FALSE ("Fl. Triggered...")
                    n1485 = local write "Fl. Triggered..."(w1947) -> ()
                    n1486 = property on="Green Laser ON/Interlacing" class="Bool (strict)"("Val(Sgnl)"=w1947) -> ()  [unwired: 2 in, 2 out]
                  }
                }
              }
            }
            n1487 = local read "Time tether formed"() -> (w1938:timestamp)
            n1488 = Get Date/Time In Seconds() -> (seconds since 1Jan1904=w1939:timestamp)
            n1489 = Subtract(x=w1939, y=w1938) -> (x-y=w1937:dbl)
            n1490 = Number To Decimal String(number=w1937) -> (decimal integer string=w1934:string)  [unwired: 1 out]
            n1491 = local read "Messages"() -> (w1941:string)
            n1492 = call <vilib>:"Beep.vi"() -> ()  [unwired: 3 in, 9 out]
            n1493 = Concatenate Strings("Lost tether (" ("Message to add"), w1934, " s)." ("string")) -> (w1936:string)
            n1494 = local write "Tether"(FALSE ("Tether")) -> ()
            n1495 = call "Update messages.vi"("Message to add"=w1936, "Old message string"=w1941) -> ("New message string"=w1940:string)
            n1496 = local write "Messages"(w1940) -> ()
            n1497 = property on="Fl. Triggered..." class="Bool (strict)"("Val(Sgnl)"=w1932) -> ()  [unwired: 2 in, 2 out]
            n1498 = local write "Dip for Protein"(w1932) -> ()
            n1499 = property on="Trap Pos. FB ON" class="Bool (strict)"("Val(Sgnl)"=w1932) -> ()  [unwired: 2 in, 2 out]
            n1500 = property on="Trap Trig. Fl." class="Bool (strict)"("Val(Sgnl)"=w1932) -> ()  [unwired: 2 in, 2 out]
          }
        }
      }
    }
    n1501 = case "For triggering actions based on the trap position (e.g., turning the excitation laser on if trap under feedback moves so far)" shown="True" "Trap Trig. Fl." {
      tunnel: w1464 -> [_ w1820]
      tunnel: w1477 -> [_ w1819]
      tunnel: ["" ("t") w1818] -> w1485
      tunnel: w1469 -> [_ w1817]
      tunnel: [0 ("t") w1816] -> w1482
      tunnel: w1481 -> [_ w1815]
      tunnel: w1456 -> [_ w1814]
      tunnel: w1455 -> [_ w1813]
      frame False {
      }
      frame True {
        n1502 = case shown="\"Wait for trigger\"" w1819 {
          tunnel: w1820 -> [w1837 _ _ w1885]
          tunnel: [w1834 w1866 "" ("t") w1888] -> w1818
          tunnel: w1817 -> [_ _ _ w1876]
          tunnel: [w1833 w1863 0 ("t") w1877] -> w1816
          tunnel: w1815 -> [_ w1865 _ w1883]
          tunnel: w1814 -> [w1822 w1860 _ w1879]
          tunnel: w1813 -> [w1821 w1859 _ w1878]
          frame "Wait for trigger" {
            n1503 = local read "Trap Trig. (FPGA)"() -> (w1825:bool)
            n1504 = Subtract(x=w1837, y="Mean T1 Position\nto compare (nm)") -> (x-y=w1830:dbl[])
            n1505 = call <vilib>:"Std Deviation and Variance.vi"("X"=w1830) -> ("mean"=→"mean":dbl, "standard deviation"=→"standard\ndeviation":dbl)  [unwired: 1 in, 1 out]
            n1506 = Array Max & Min(array=w1830) -> (max value=→"max value":dbl, min value=→"min value":dbl)  [unwired: 2 out]
            n1507 = Greater?(x=w1830, y="Threshold (nm)") -> (0:w1840:bool[])
            n1508 = case shown="True" w1825 {
              tunnel: w1822 -> [_ w1846]
              tunnel: w1821 -> [_ w1845]
              tunnel: [FALSE ("TTrig?") w1844] -> w1828
              frame False {
              }
              frame True {
                n1509 = xnode "Read/Write Control"("FPGA VI Reference In"=w1846, "error in"=w1845) -> ("TTrig?"=w1844:bool)  [unwired: 2 out]
              }
            }
            n1510 = Or Array Elements(Boolean array=w1840) -> (logical OR=w1827:bool)
            n1511 = Select(t=w1828, s=w1825, f=w1827) -> (s? t:f=w1826:bool)
            n1512 = Not(x=w1825) -> (.not. x?=w1824:bool)
            n1513 = And(x=w1826, y=w1824) -> (x .and. y?=w1823:bool)
            n1514 = Select(t="Triggered", s=w1826, f="Wait for trigger") -> (s? t:f=w1834:string)
            n1515 = case shown="True" w1826 {
              tunnel: [0 0] -> w1833
              tunnel: w1822 -> [_ w1851]
              tunnel: w1821 -> [_ w1850]
              frame False {
                "Waiting" <- TRUE ("Waiting")
              }
              frame True {
                n1516 = xnode "Read/Write Control"("FPGA VI Reference In"=w1851, "error in"=w1850, "TTrig?"=FALSE) -> ()  [unwired: 2 out]
                n1517 = local read "Messages"() -> (w1854:string)
                n1518 = call <vilib>:"Beep.vi"() -> ()  [unwired: 12 in]
                n1519 = call "Update messages.vi"("Message to add"="Unwinding trigger.", "Old message string"=w1854) -> ("New message string"=w1855:string)
                n1520 = local write "Messages"(w1855) -> ()
                n1521 = local write "Waiting"(FALSE ("Waiting")) -> ()
                "Triggered" <- TRUE ("Triggered")
              }
            }
            n1522 = case "Only need to turn on laser if host triggered" shown="True" w1823 {
              frame False {
              }
              frame True {
                n1523 = property on="Green Laser ON/Interlacing" class="Bool (strict)"("Val(Sgnl)"=TRUE ("Value (Signaling)")) -> ()  [unwired: 2 in, 2 out]
              }
            }
          }
          frame "Triggered" {
            n1524 = local read "Trap Trig. (FPGA)"() -> (w1862:bool)
            n1525 = Increment(x=w1865) -> (x+1=w1863:i32)
            n1526 = Greater Or Equal?(x=w1863, y="Fl. ON time (n)") -> (x >= y?=w1861:bool)
            n1527 = Select(t="Wait for trigger", s=w1861, f="Triggered" ("t")) -> (s? t:f=w1866:string)
            n1528 = And(x=w1861, y=w1862) -> (x .and. y?=w1858:bool)
            n1529 = case shown="True" w1858 {
              tunnel: w1860 -> [_ w1870]
              tunnel: w1859 -> [_ w1869]
              frame False {
              }
              frame True {
                n1530 = xnode "Read/Write Control"("FPGA VI Reference In"=w1870, "error in"=w1869, "FPGA Trap Trig"=TRUE) -> ()  [unwired: 2 out]
              }
            }
            n1531 = case shown="True" w1861 {
              frame False {
              }
              frame True {
                w1872 = FALSE ("Value (Signaling)")
                n1532 = local write "Triggered"(w1872) -> ()
                n1533 = local write "Waiting"(TRUE ("Waiting")) -> ()
                n1534 = property on="Green Laser ON/Interlacing" class="Bool (strict)"("Val(Sgnl)"=w1872) -> ()  [unwired: 2 in, 2 out]
              }
            }
          }
          frame "Do nothing" {
          }
          frame "Initialize", Default {
            n1535 = Increment(x=w1883) -> (x+1=w1887:i32)
            n1536 = Select(t=1, s=w1876, f=w1887) -> (s? t:f=w1877:i32)
            n1537 = feedback #27(w1885) -> (w1891:dbl[])
            n1538 = Build Array (concatenate)(w1885, w1891) -> (w1884:dbl[])
            n1539 = Greater Or Equal?(x=w1877, y="Wait to get offset (n)") -> (x >= y?=w1880:bool)
            n1540 = Select(t=w1885, s=w1876, f=w1884) -> (s? t:f=w1886:dbl[])
            n1541 = feedback-in #27(w1886) -> ()
            n1542 = call-poly <vilib>:"Mean.vi"("X"=w1886) -> ("mean"=w1881:dbl)  [unwired: 1 out]
            n1543 = local write "Mean T1 Position\nto compare (nm)"(w1881) -> ()
            n1544 = case shown="True" w1876 {
              tunnel: w1879 -> [_ w1897]
              tunnel: w1878 -> [_ w1896]
              frame False {
              }
              frame True {
                w1893 = FALSE ("FPGA Trap Trig")
                n1545 = xnode "Read/Write Control"("FPGA VI Reference In"=w1897, "error in"=w1896, "FPGA Trap Trig"=w1893) -> ("FPGA VI Reference Out"=w1895:T20, "error out"=w1894:errorcluster)
                n1546 = xnode "Read/Write Control"("FPGA VI Reference In"=w1895, "error in"=w1894, "TTrig?"=w1893) -> ()  [unwired: 2 out]
              }
            }
            n1547 = Select(t="Wait for trigger", s=w1880, f="Initialize") -> (s? t:f=w1888:string)
            n1548 = case shown="True" w1880 {
              tunnel: w1881 -> [_ w1900]
              tunnel: w1879 -> [_ w1909]
              tunnel: w1878 -> [_ w1908]
              frame False {
                n1549 = local write "Waiting"(FALSE ("Waiting")) -> ()
                "Initializing" <- TRUE ("Initializing")
              }
              frame True {
                n1550 = local read "Threshold (nm)"() -> (w1912:dbl)
                n1551 = local read "AOM X Cal (nm/MHz)"() -> (w1911:dbl)
                n1552 = Add(x=w1900, y=w1912) -> (x+y=w1913:dbl)
                n1553 = Divide(x=w1913, y=w1911) -> (x/y=w1910:dbl)
                n1554 = call "IR AOM freq to word.vi"("Frequency In (MHz)"=w1910) -> ("Frequency Word Out (double)"=w1907:dbl)
                n1555 = local write "Initializing"(FALSE ("Initializing")) -> ()
                n1556 = local write "Waiting"(TRUE ("Waiting")) -> ()
                n1557 = To Quad Integer(1:w1907) -> (0:w1906:i64)
                n1558 = xnode "Read/Write Control"("FPGA VI Reference In"=w1909, "error in"=w1908, "FPGA TTrig Thresh"=w1906) -> ("FPGA VI Reference Out"=w1903:T20, "error out"=w1902:errorcluster)
                n1559 = xnode "Read/Write Control"("FPGA VI Reference In"=w1903, "error in"=w1902, "FPGA Trap Trig"=TRUE) -> ()  [unwired: 2 out]
              }
            }
          }
        }
      }
    }
    n1560 = feedback-in #24(w1485) -> ()
    n1561 = feedback-in #25(w1482) -> ()
    n1562 = Split 1D Array(array=w1437, index=w1499) -> (first subarray=w1609:dbl[])  [unwired: 1 out]
    n1563 = feedback-in #26(w1609) -> ()
    n1564 = call-poly <vilib>:"Mean.vi"("X"=w1609) -> ("mean"=w1608:dbl)  [unwired: 1 out]
    "Bead Mean (nm)" <- w1608
    n1565 = Subtract(x=w1609, y=w1608) -> (x-y=w1607:dbl[])
    n1566 = Square(x=w1607) -> (x^2=w1606:dbl[])
    n1567 = call-poly <vilib>:"Mean.vi"("X"=w1606) -> ("mean"=w1605:dbl)  [unwired: 1 out]
    n1568 = Square Root(x=w1605) -> (sqrt(x)=w1604:dbl)
    n1569 = Multiply(x=10.0, y=w1604) -> (x*y=→"RMS (Ang)":dbl)
    n1570 = xnode ("Read/Write Control")("FPGA VI Reference In"=w1642, "error in"=w1641) -> ("FPGA VI Reference Out"=w1467:T20, "error out"=w1466:errorcluster, "AI2 Y Sum Set 1"=w1748:i16, "AI2 Y Sum Set 2"=w1747:i16, "AI1 X Set 1"=w1531:fxp<+/-,16,1>, "AI1 X Set 2"=w1530:fxp<+/-,16,1>, "Trap Pos FB Int Signal"=→"Trap Pos FB Int Signal":fxp<+/-,24,9>, "Trap Pos FB Int-Norm Signal"=→"Trap Pos FB Int-Norm Signal":fxp<+/-,16,1>, "Trap Pos FB Action"=w1524:i64, "Scanning"=→"AOD Scanning":bool, "Scan I"=→"AOD Scan I":u64, "Scanning MCL"=w1750:bool, "Scan I (MCL)"=→"MCL Scan I":u64, "Green FB Signals"=w1687:T45, "Trap Pos FB Action"=w1454:i64, "TTrig Fin Thresh"=w1450:i64)
    "MCL Scanning" <- w1750
    "Trap Pos FB Action" <- w1524
    n1571 = local read "FB Trig Integrate"() -> (w1448:u32)
    n1572 = Divide(x=w1454, y=w1448) -> (x/y=w1447:dbl)
    "TTrig Sig (Int)" <- w1447
    n1573 = Divide(x=w1450, y=w1448) -> (x/y=w1445:dbl)
    "TTrig Fin Thresh (Int)" <- w1445
    n1574 = local read "AOM X Cal (nm/MHz)"() -> (w1453:dbl)
    n1575 = local read "AI2 (V)"() -> (w1749:cluster{"Set 1":dbl, "Set 2":dbl})
    n1576 = Bundle By Name(cluster=w1749, "Set 1"=w1748, "Set 2"=w1747) -> (w1745:cluster{"Set 1":dbl, "Set 2":dbl})
    n1577 = Divide(x=w1524, y=327.67) -> (x/y=→"Action (%)":dbl)
    n1578 = local read "Trap X (AI1)"() -> (w1544:T11)
    n1579 = call "IR AOM word double to freq.vi"("Frequency Word In (double)"=w1445) -> ("Frequency Out (MHz)"=w1444:dbl)
    n1580 = call "IR AOM word double to freq.vi"("Frequency Word In (double)"=w1447) -> ("Frequency Out (MHz)"=w1446:dbl)
    n1581 = Divide(x=w1745, y=3276.7) -> (x/y=w1744:cluster{"Set 1":dbl, "Set 2":dbl})
    n1582 = Multiply(x=w1446, y=w1453) -> (x*y=w1452:dbl)
    "TTrig Sig (nm)" <- w1452
    n1583 = Multiply(x=w1444, y=w1453) -> (x*y=w1451:dbl)
    "TTrig Fin Thresh (nm)" <- w1451
    n1584 = local write "AI2 (V)"(w1744) -> ()
    n1585 = Bundle(cluster=w1544, "Trap 1"=w1531, "Trap 2"=w1530) -> (→"Trap X (AI1)":T11)
    n1586 = Bundle(w1452, w1451) -> (→"TTrig":cluster{dbl, dbl})  [unwired: 1 in]
    n1587 = Divide(x=w1687, y=3276.7) -> (x/y=w1683:T46)
    n1588 = Unbundle By Name(w1683) -> ("Green FB Ch 0"=w1686:dbl, "Green FB Ch 1"=w1685:dbl, "Green FB Ch 2"=w1684:dbl)
    n1589 = Divide(x=w1686, y=w1684) -> (x/y=w1682:dbl)
    n1590 = Divide(x=w1685, y=w1684) -> (x/y=w1681:dbl)
    n1591 = flat-sequence "To save data" {
      tunnel: [w2768] -> w1767
      tunnel: [w2769] -> w1766
      tunnel: w1718 -> [w2762]
      tunnel: w1472 -> [w2766]
      tunnel: ["Save Calibration"] -> w1741
      tunnel: w1738 -> [w2765]
      tunnel: [w2758] -> w1737
      tunnel: [w2755] -> w1736
      tunnel: [w2752] -> w1735
      tunnel: w1717 -> [w2754]
      tunnel: w1624 -> [w2748]
      tunnel: [w2748] -> w1623
      tunnel: ["Start Saving"] -> w1589
      tunnel: [w2742] -> w1512
      tunnel: [w2741] -> w1511
      tunnel: w1767 -> [w3015]
      tunnel: w1766 -> [w3014]
      tunnel: w1513 -> [w3013]
      tunnel: w1741 -> [w3012]
      tunnel: w1737 -> [w3010]
      tunnel: w1736 -> [w3009]
      tunnel: w1735 -> [w3008]
      tunnel: w1598 -> [w3007]
      tunnel: w1634 -> [w3006]
      tunnel: w1623 -> [w3005]
      tunnel: w1589 -> [w3004]
      tunnel: w1587 -> [w3003]
